vi "IMAGE TO BITS.vi"() -> ()   [LabVIEW 2013]
panel:
  out "VHDL":string
  out "Y":i32
  out "X":i32
  out "new picture":picture
  out "Array":string[][](array[string])
  in  "Path":path=path "C:/VIVADO_PROJECTS/VLAK/00GRAPHICS/TEST2.png"
  # "feed PNG picture 24bit color depth without transparency"
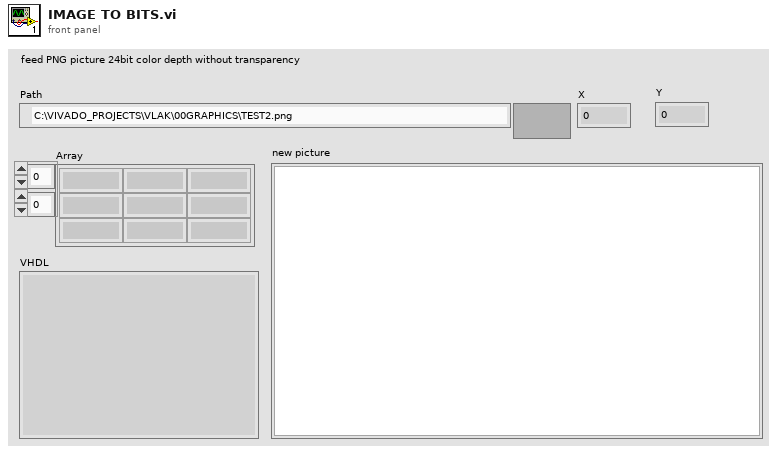
[diagram p1: front panel]
types:
  T1 = typedef "imagedata.ctl" = cluster{"image type":i32, "image depth":i32, "image":u8[], "mask":u8[], "colors":u32[], "Rectangle":cluster{"left":i16, "top":i16, "right":i16, "bottom":i16}}
  T2 = cluster{"left":i16, "top":i16, "right":i16, "bottom":i16}
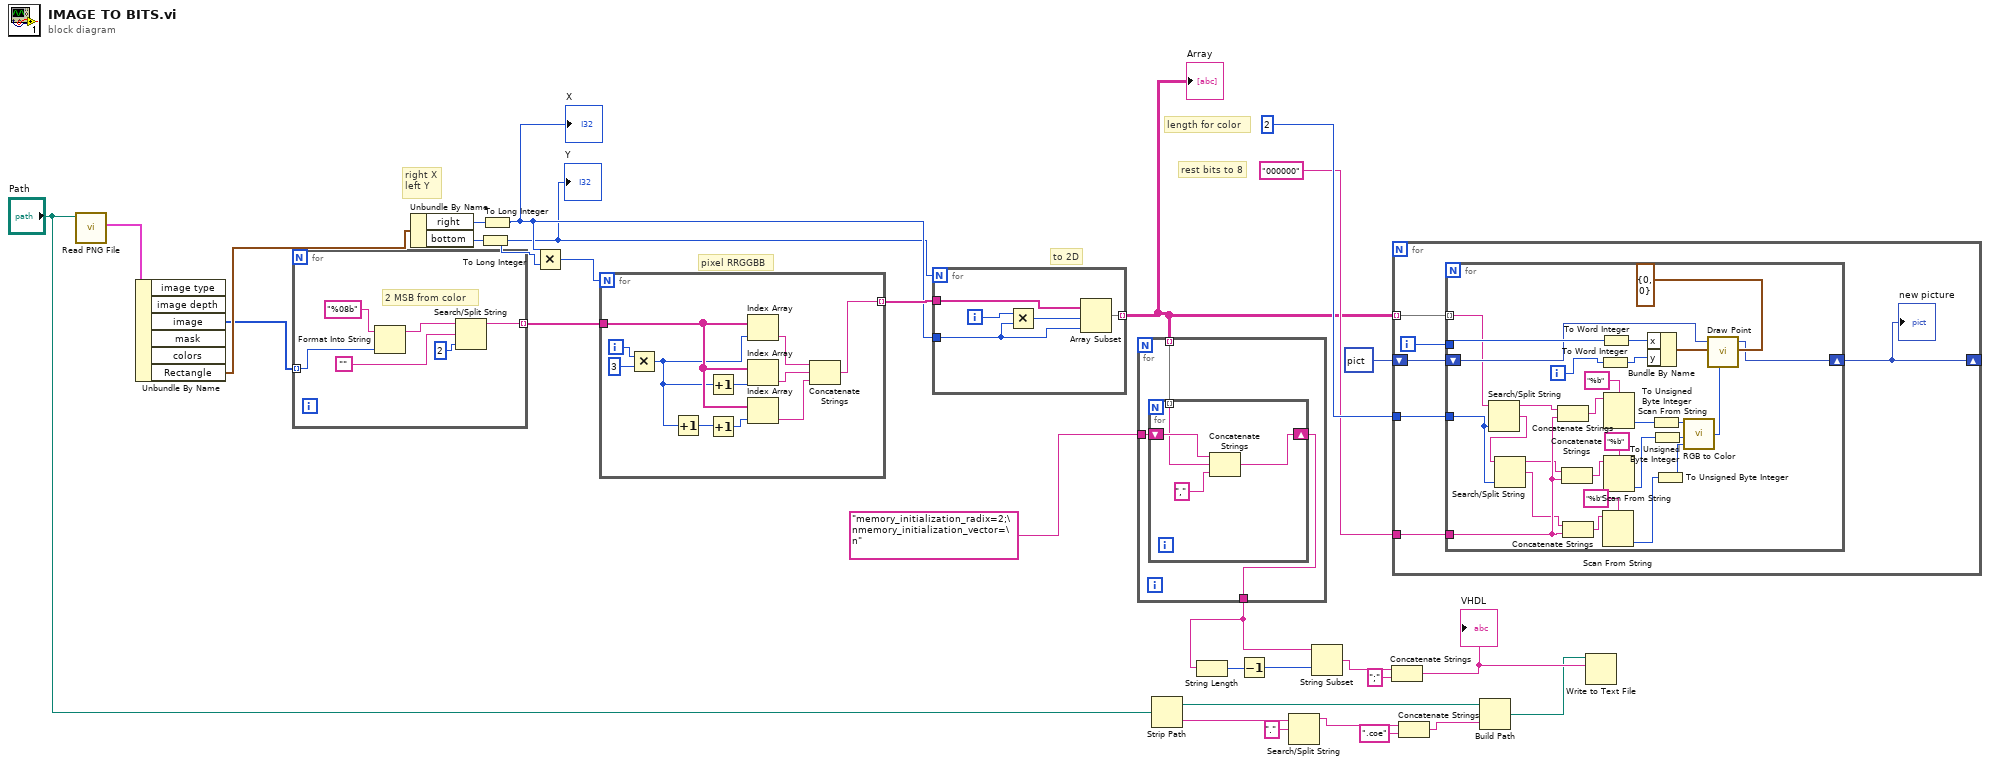
[diagram p0: block diagram]
diagram:
  # "rest bits to 8"
  # "length for color"
  # "right X\nleft Y"
  # "pixel RRGGBB"
  # "to 2D"
  n1 = call <vilib>:"Read PNG File.vi"("path to PNG file"="Path") -> ("image data"=w29:T1)  [unwired: 8 in, 2 out]
  n2 = Unbundle By Name(w29) -> ("image"=w27:u8[], "Rectangle"=w28:T2)  [unwired: 4 out]
  n3 = for {
    tunnel: w27 -> [w34] mode=indexing
    tunnel: [w30] -> w26 mode=indexing
    # "2 MSB from color"
    n4 = Format Into String(format string="%08b", w34) -> (resulting string=w33:string)  [unwired: 2 in, 1 out]
    n5 = Search/Split String(string=w33, search string/char (-)="", offset (0)=2) -> (substring before match=w30:string)  [unwired: 2 out]
  }
  n6 = Unbundle By Name(w28) -> ("right"=w23:i16, "bottom"=w24:i16)
  n7 = To Long Integer(number=w24) -> (32bit integer=w18:i32)
  "Y" <- w18
  n8 = To Long Integer(number=w23) -> (32bit integer=w19:i32)
  "X" <- w19
  n9 = Multiply(x=w19, y=w18) -> (x*y=w4:i32)
  n10 = for {
    N: w4 -> [_]
    tunnel: w26 -> [w46]
    tunnel: [w36] -> w25 mode=indexing
    i -> [w42]
    n11 = Multiply(x=w42, y=3) -> (x*y=w38:i32)
    n12 = Increment(x=w38) -> (x+1=w37:i32)
    n13 = Increment(x=w38) -> (x+1=w40:i32)
    n14 = Increment(x=w37) -> (x+1=w39:i32)
    n15 = Index Array(array=w46, index=w38) -> (element=w45:string)
    n16 = Index Array(array=w46, index=w40) -> (element=w44:string)
    n17 = Index Array(array=w46, index=w39) -> (element=w43:string)
    n18 = Concatenate Strings(w45, w44, w43) -> (w36:string)
  }
  n19 = for {
    N: w18 -> [_]
    tunnel: w19 -> [w51]
    tunnel: w25 -> [w48]
    tunnel: [w47] -> w17 mode=indexing
    i -> [w50]
    n20 = Multiply(x=w50, y=w51) -> (x*y=w49:i32)
    n21 = Array Subset(array=w48, index=w49, length=w51) -> (w47:string[])
  }
  "Array" <- w17
  n22 = for {
    tunnel: w17 -> [w54] mode=indexing
    tunnel: "memory_initialization_radix=2;\nmemory_initialization_vector=\n" ("string") -> [w53]
    tunnel: [w52] -> w1
    n23 = for {
      tunnel: w54 -> [w56] mode=indexing
      shift-right: [w57] -> w52
      shift-left: w53 -> [w58]
      n24 = Concatenate Strings(w58, w56, "," ("string")) -> (w57:string)
    }
  }
  n25 = Strip Path(path="Path") -> (stripped path=w11:path, name=w10:string)
  n26 = String Length(string=w1) -> (length=w3:i32)
  n27 = Decrement(x=w3) -> (x-1=w2:i32)
  n28 = Search/Split String(string=w10, search string/char (-)=".") -> (substring before match=w8:string)  [unwired: 1 in, 2 out]
  n29 = String Subset(string=w1, length (rest)=w2) -> (substring=w14:string)  [unwired: 1 in]
  n30 = Concatenate Strings(w14, ";" ("string")) -> (w12:string)
  "VHDL" <- w12
  n31 = for {
    tunnel: w17 -> [w64] mode=indexing
    shift-right: [w62] -> _
    shift-left: picture data[5B] ("new picture") -> [w61]
    tunnel: 2 ("index") -> [w60]
    tunnel: "000000" ("string") -> [w59]
    i -> [w63]
    n32 = for {
      tunnel: w64 -> [w74] mode=indexing
      tunnel: w63 -> [w87]
      shift-right: [w85] -> w62
      shift-left: w61 -> [w84]
      tunnel: w60 -> [w72]
      tunnel: w59 -> [w71]
      i -> [w86]
      n33 = Search/Split String(string=w74, offset (0)=w72) -> (substring before match=w70:string, match + rest of string=w73:string)  [unwired: 1 in, 1 out]
      n34 = Search/Split String(string=w73, offset (0)=w72) -> (substring before match=w68:string, match + rest of string=w66:string)  [unwired: 1 in, 1 out]
      n35 = Concatenate Strings(w70, w71) -> (w69:string)
      n36 = Concatenate Strings(w68, w71) -> (w67:string)
      n37 = Concatenate Strings(w66, w71) -> (w65:string)
      n38 = To Word Integer(number=w86) -> (16bit integer=w89:i16)
      n39 = To Word Integer(number=w87) -> (16bit integer=w88:i16)
      n40 = Scan From String(format string="%b", input string=w65) -> (output 1=w75:i32)  [unwired: 3 in, 3 out]
      n41 = Scan From String(format string="%b", input string=w69) -> (output 1=w79:i32)  [unwired: 3 in, 3 out]
      n42 = Scan From String(format string="%b", input string=w67) -> (output 1=w76:i32)  [unwired: 3 in, 3 out]
      n43 = Bundle By Name(cluster=cluster{"y":i16, "x":i16} {"y"=0, "x"=0} ("point(x,y)"), "x"=w88, "y"=w89) -> (w90:cluster{"y":i16, "x":i16})
      n44 = To Unsigned Byte Integer(number=w79) -> (unsigned 8bit integer=w82:u8)
      n45 = To Unsigned Byte Integer(number=w76) -> (unsigned 8bit integer=w80:u8)
      n46 = To Unsigned Byte Integer(number=w75) -> (unsigned 8bit integer=w81:u8)
      n47 = call <vilib>:"RGB to Color.vi"("B"=w81, "G"=w80, "R"=w82) -> ("Color"=w92:u32)
      n48 = call <vilib>:"Draw Point.vi"("picture"=w84, "point(x,y)"=w90, "color(black)"=w92) -> ("new picture"=w85:picture)  [unwired: 6 in]
    }
    "new picture" <- w62
  }
  n49 = Concatenate Strings(w8, ".coe" ("string")) -> (w6:string)
  n50 = Build Path(base path=w11, name or relative path=w6) -> (appended path=w5:path)
  n51 = Write to Text File(file (use dialog)=w5, text=w12) -> ()  [unwired: 2 in, 3 out]
